vi "OCR Check(Center & Left).vi"(8 "error in (no error)":errorcluster, 11 "Image Path":path=path "C:/images/img1.jpeg") -> (0 "error out":errorcluster, 1 "Image Out":T2(plugin-control), 2 "RIGHT":bool, 3 "OCR Check":T3={"C_Center"="6 G D 6 4 8 6", "Center 2"=TRUE, "C_Top"="8 G D 6 4 8 6", "Top 2"=TRUE, "C_Bottom"="6 G D 6 4 4 8", "Bottom 2"=TRUE, "RH_TOP"="", "Top_RH"=FALSE, "RH_CENTER"="", "Center_RH"=FALSE, "RH_BOTTOM"="6 G D 6 4 8 6", "Bottom_RH"=TRUE}, 7 "Pattern Presence":bool)   [LabVIEW 2019]
panel:
  out "OCR 3 Digit":T1
  out "CENTER":bool
  out "Read bottom":string
  out "Read Center":string caption="Read String"
  out "Read Top":string
  out "y":sgl=319.5874
  out "x":sgl=660.16455
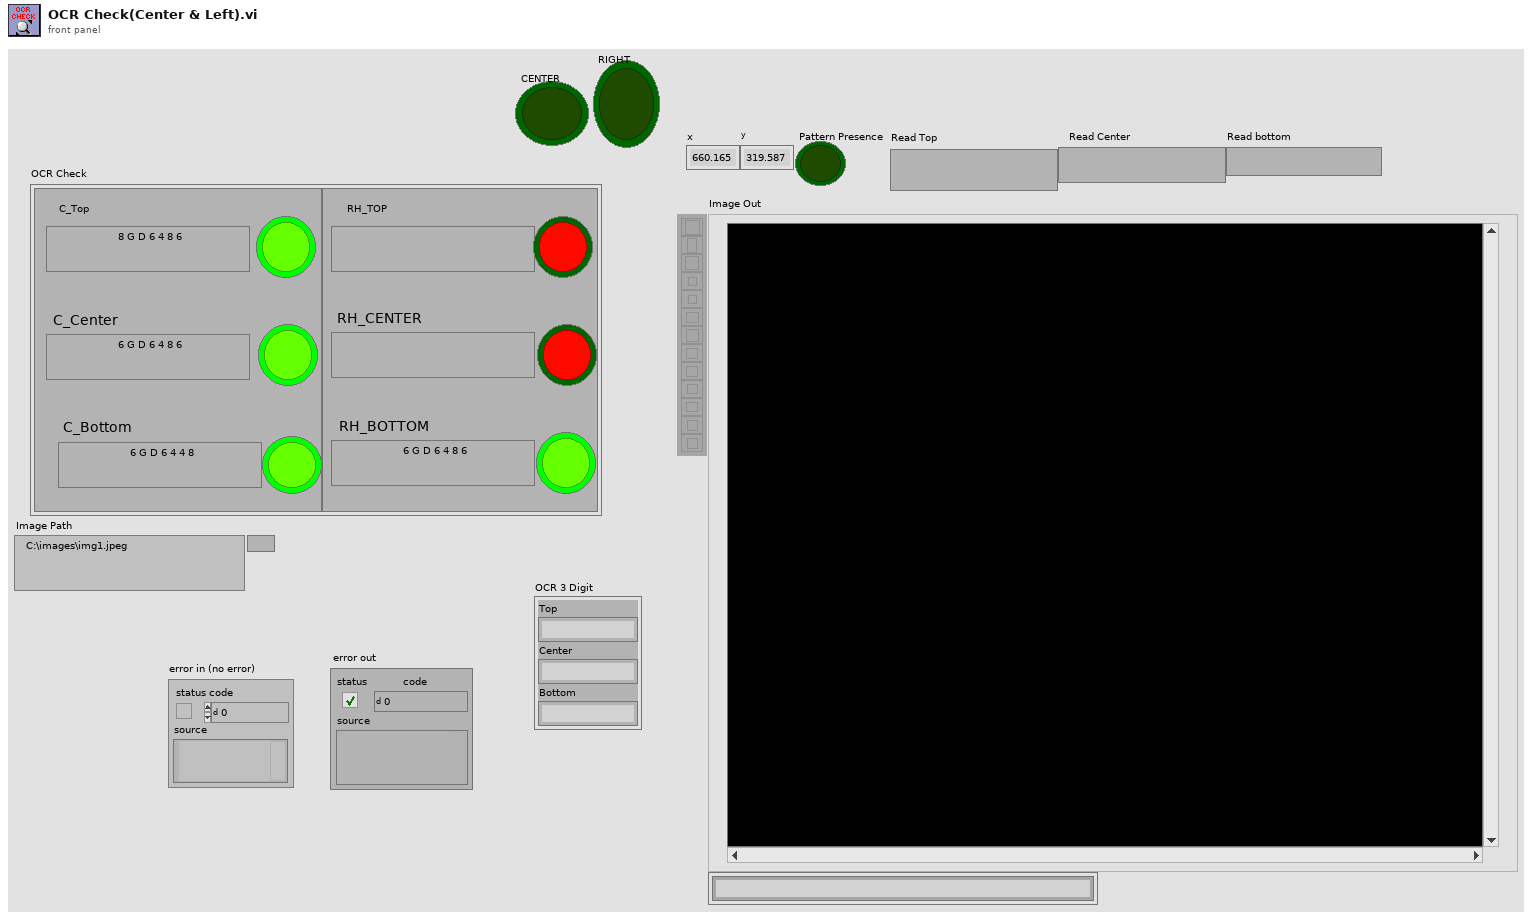
[diagram p1: front panel]
types:
  T1 = cluster{"Top":string, "Center":string, "Bottom":string}
  T2 = typedef "IMAQ Image.ctl" = refnum<image>
  T3 = cluster{"C_Center":string, "Center 2":bool, "C_Top":string, "Top 2":bool, "C_Bottom":string, "Bottom 2":bool, "RH_TOP":string, "Top_RH":bool, "RH_CENTER":string, "Center_RH":bool, "RH_BOTTOM":string, "Bottom_RH":bool}
  T4 = cluster{"Center":string, "Center 2":bool, "Top":string, "Top 2":bool, "Bottom":string, "Bottom 2":bool, "RH_TOP":string, "Top_RH":bool, "RH_CENTER":string, "Center_RH":bool, "RH_BOTTOM":string, "Bottom_RH":bool}
  T5 = typedef "Image Type" = u32
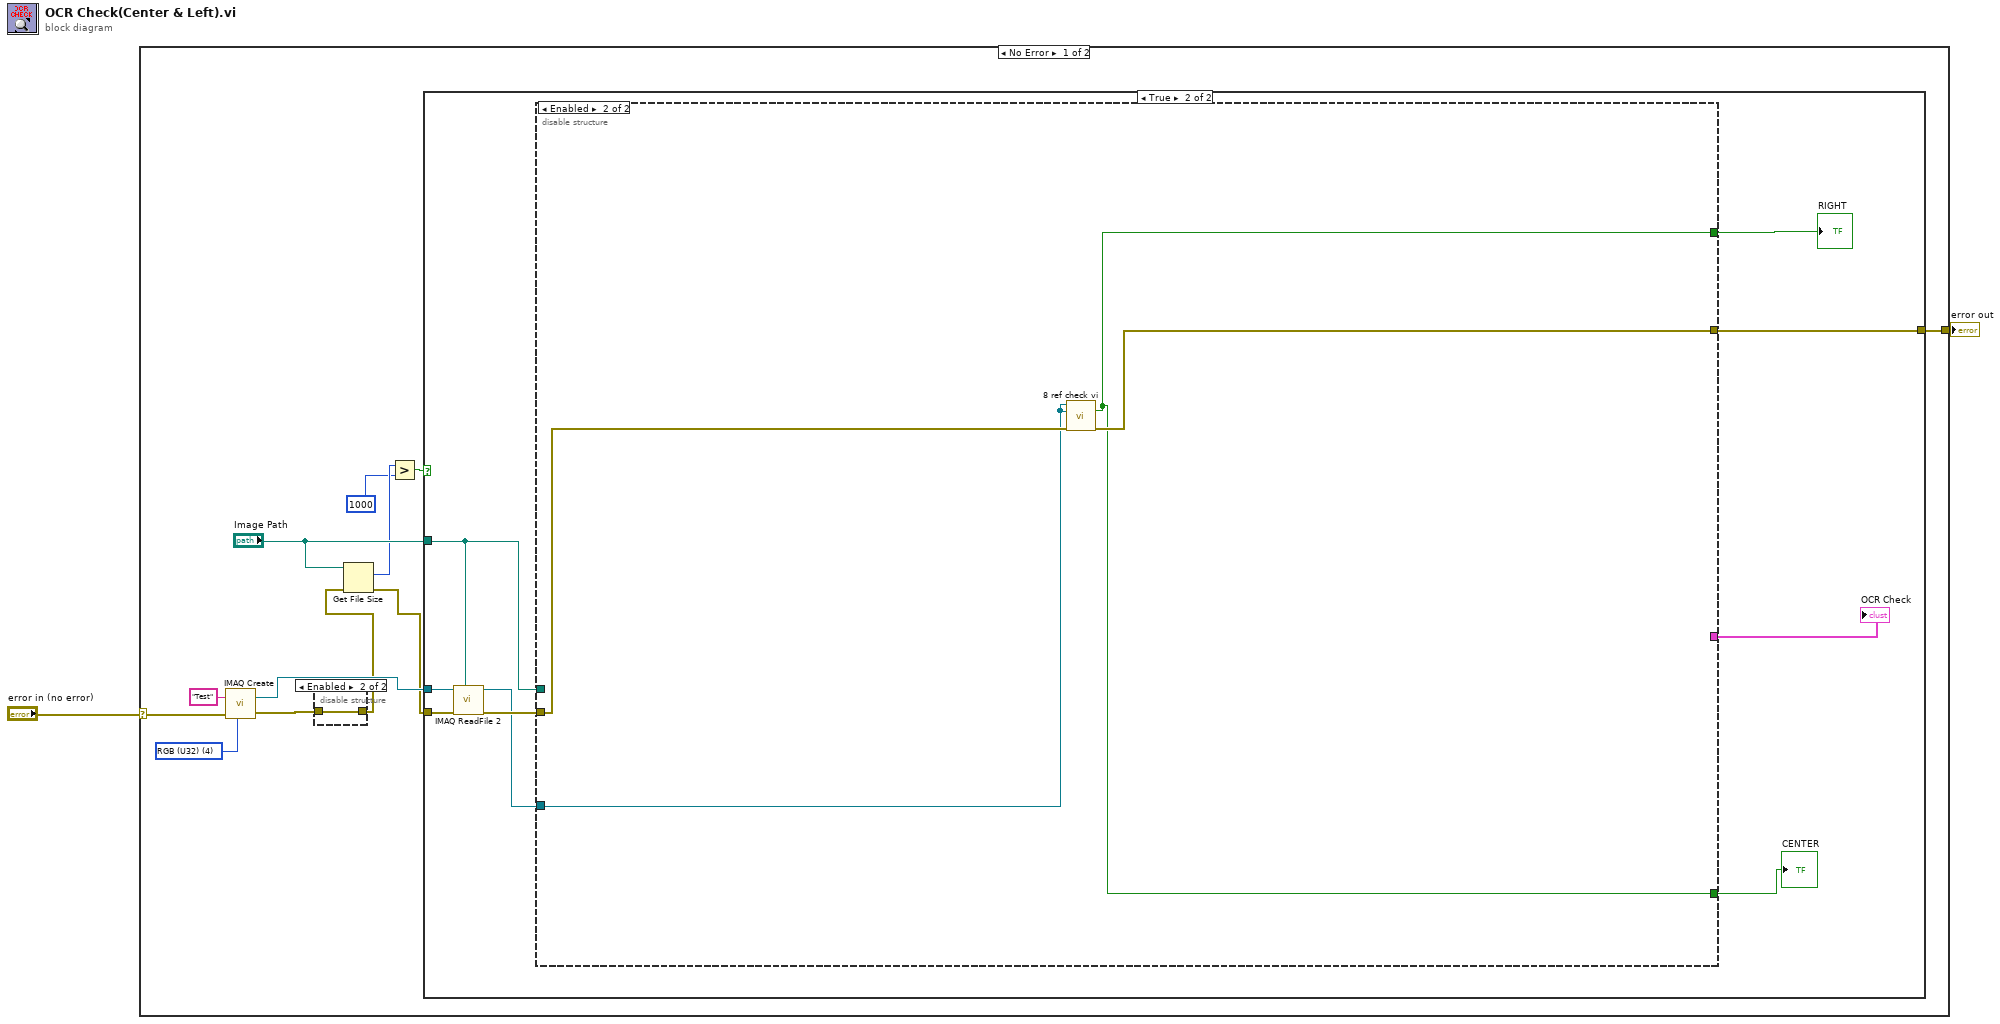
[diagram p0: block diagram]
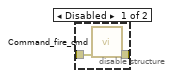
[diagram p2: hidden frame]
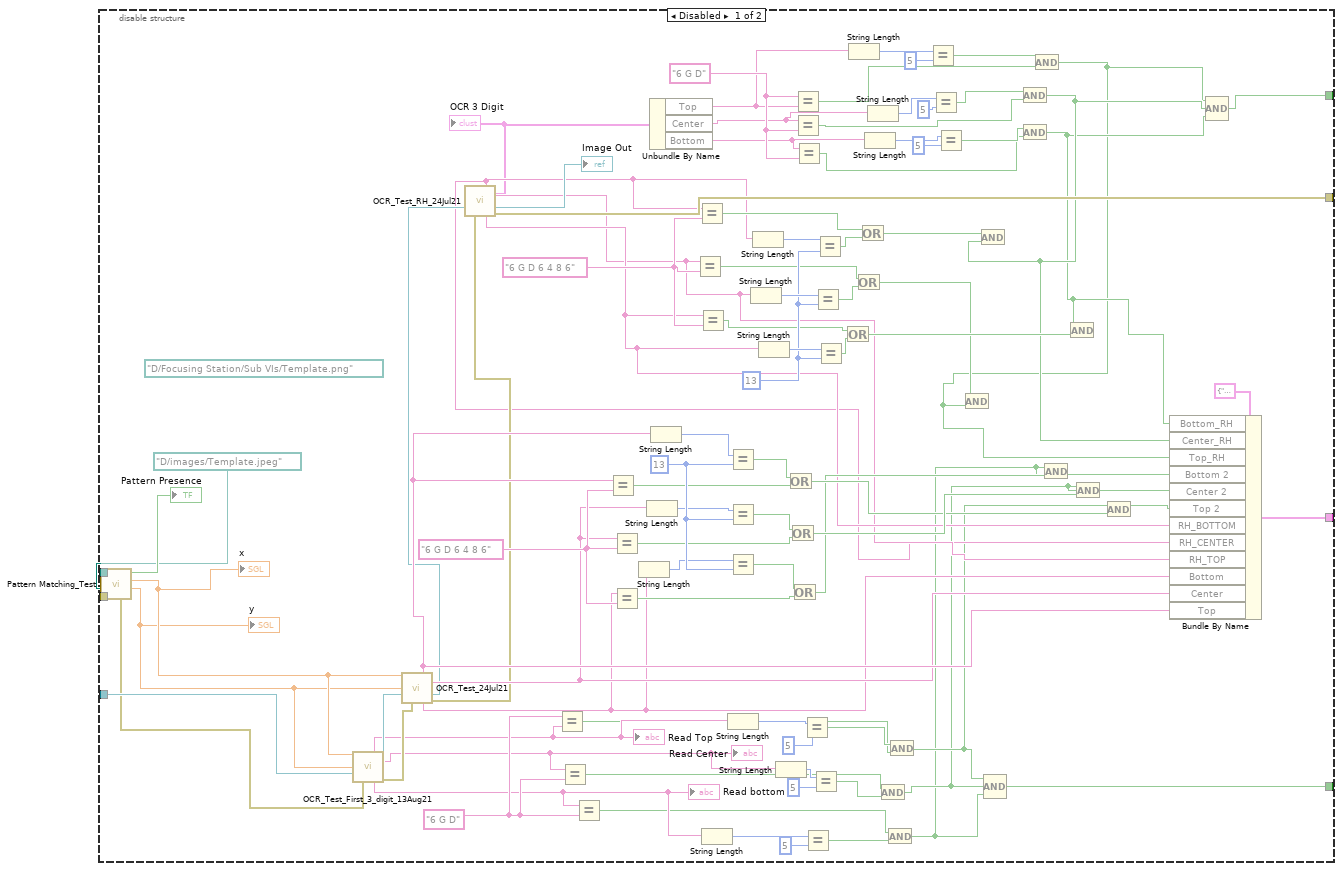
[diagram p4: hidden frame]
diagram:
  n1 = case shown="No Error" "error in (no error)" {
    selector: "error in (no error)" -> [w3 w123]
    tunnel: [w4 w123] -> w2
    frame No Error {
      w12 = T5 4 items=["Grayscale (U8)", "Grayscale (I16)", "Grayscale (SGL)", "Complex (CSG)", "RGB (U32)", "HSL (U32)", "RGB (U64)", "Grayscale (U16)"] ("Image Type")
      n2 = call "IMAQ Create"("Image Name"="Test", "Image Type"=w12, "error in (no error)"=w3) -> ("New Image"=w14:T2, "error out"=w11:errorcluster)  [unwired: 2 in]
      n3 = disable-structure shown="Enabled" {
        disable-tunnel: w11 -> [w16 w17]
        disable-tunnel: [w15 w17] -> w8
        frame Disabled {
          n4 = call "Command_fire_cmd.vi"("error in"=w16) -> ("error out"=w15:errorcluster)  [unwired: 6 in, 2 out]
        }
        frame Enabled {
        }
      }
      n5 = Get File Size(file="Image Path", error in=w8) -> (size (in bytes)=w7:i64, 0:w9:errorcluster)  [unwired: 1 out]
      n6 = Greater?(x=w7, y=i64 1000) -> (0:w5:bool)
      n7 = case shown="True" w5 {
        tunnel: w14 -> [_ w26]
        tunnel: "Image Path" -> [_ w24]
        tunnel: w9 -> [w18 w23]
        tunnel: [w18 w22] -> w4
        frame False {
        }
        frame True {
          n8 = call "IMAQ ReadFile 2"("File Path"=w24, "error in (no error)"=w23, "Image"=w26) -> ("error out"=w25:errorcluster, "Image Out"=w21:T2)  [unwired: 4 in, 3 out]
          n9 = disable-structure shown="Enabled" {
            disable-tunnel: [w87 _] -> w27
            disable-tunnel: w25 -> [w83 w121]
            disable-tunnel: w24 -> [w82 _]
            disable-tunnel: [w80 w122] -> w22
            disable-tunnel: w21 -> [w72 w119]
            disable-tunnel: [w29 w120] -> w20
            disable-tunnel: [w28 w120] -> w19
            frame Disabled {
              (unwired) path "D:/Focusing Station/Sub VIs/Template.png" ("Image File Path")
              w51 = "6 G D" ("y")
              w68 = "6 G D" ("y")
              w103 = 13
              w117 = 13 ("y")
              w104 = "6 G D 6 4 8 6" ("y")
              w118 = "6 G D 6 4 8 6" ("y")
              n10 = call "Pattern Matching_Test.vi"("error in (no error)"=w83, "Template file path"=path "D:/images/Template.jpeg" ("Image File Path"), "File Path"=w82) -> ("y"=w73:sgl, "x"=w74:sgl, "Pattern Presence"=→"Pattern Presence":bool, "error out"=w70:errorcluster)  [unwired: 4 in, 1 out]
              "x" <- w74
              "y" <- w73
              n11 = call "OCR_Test_First_3_digit_13Aug21.vi"("x"=w74, "y"=w73, "Image in"=w72, "error in (no error)"=w70) -> ("Read Top"=w66:string, "Read Center"=w65:string, "Image"=w71:T2, "Read bottom"=w67:string, "error out"=w69:errorcluster)  [unwired: 7 in]
              "Read Top" <- w66
              "Read Center" <- w65
              "Read bottom" <- w67
              n12 = call "OCR_Test_24Jul21.vi"("x"=w74, "y"=w73, "Image in"=w71, "error in (no error)"=w69) -> ("Read Top"=w102:string, "Read Center"=w101:string, "Image"=w85:T2, "Read bottom"=w100:string, "error out"=w84:errorcluster)  [unwired: 7 in]
              n13 = call "OCR_Test_RH_24Jul21.vi"("Image in"=w85, "error in (no error)"=w84) -> ("OCR 3 Digit"=w52:T1, "Read Center"=w77:string, "Read Top"=w78:string, "Image"=→"Image Out":T2, "Read bottom"=w96:string, "error out"=w80:errorcluster)  [unwired: 8 in]
              "OCR 3 Digit" <- w52
              n14 = Equal?(x=w68, y=w66) -> (x = y?=w57:bool)
              n15 = Equal?(x=w65, y=w68) -> (x = y?=w54:bool)
              n16 = Equal?(x=w67, y=w68) -> (x = y?=w56:bool)
              n17 = Equal?(x=w102, y=w118) -> (x = y?=w116:bool)
              n18 = Equal?(x=w101, y=w118) -> (x = y?=w111:bool)
              n19 = Equal?(x=w100, y=w118) -> (x = y?=w110:bool)
              n20 = String Length(string=w100) -> (length=w112:i32)
              n21 = String Length(string=w101) -> (length=w113:i32)
              n22 = Unbundle By Name(w52) -> ("Top"=w50:string, "Center"=w49:string, "Bottom"=w48:string)
              n23 = String Length(string=w102) -> (length=w114:i32)
              n24 = Equal?(x=w78, y=w104) -> (x = y?=w93:bool)
              n25 = Equal?(x=w77, y=w104) -> (x = y?=w94:bool)
              n26 = Equal?(x=w96, y=w104) -> (x = y?=w91:bool)
              n27 = String Length(string=w67) -> (length=w64:i32)
              n28 = Equal?(x=w114, y=w117) -> (x = y?=w115:bool)
              n29 = Equal?(x=w113, y=w117) -> (x = y?=w108:bool)
              n30 = Equal?(x=w112, y=w117) -> (x = y?=w109:bool)
              n31 = String Length(string=w66) -> (length=w61:i32)
              n32 = String Length(string=w78) -> (length=w106:i32)
              n33 = String Length(string=w77) -> (length=w107:i32)
              n34 = String Length(string=w96) -> (length=w105:i32)
              n35 = String Length(string=w65) -> (length=w62:i32)
              n36 = Or(x=w115, y=w116) -> (x .or. y?=w98:bool)
              n37 = Or(x=w108, y=w111) -> (x .or. y?=w99:bool)
              n38 = Or(x=w109, y=w110) -> (x .or. y?=w97:bool)
              n39 = Equal?(x=w51, y=w50) -> (x = y?=w40:bool)
              n40 = Equal?(x=w49, y=w51) -> (x = y?=w38:bool)
              n41 = Equal?(x=w48, y=w51) -> (x = y?=w36:bool)
              n42 = Equal?(x=w61, y=5) -> (x = y?=w58:bool)
              n43 = Equal?(x=w64, y=5) -> (x = y?=w55:bool)
              n44 = Equal?(x=w62, y=5) -> (x = y?=w53:bool)
              n45 = Equal?(x=w106, y=w103) -> (x = y?=w92:bool)
              n46 = Equal?(x=w107, y=w103) -> (x = y?=w95:bool)
              n47 = Equal?(x=w105, y=w103) -> (x = y?=w90:bool)
              n48 = Or(x=w91, y=w90) -> (x .or. y?=w89:bool)
              n49 = String Length(string=w50) -> (length=w47:i32)
              n50 = Or(x=w93, y=w92) -> (x .or. y?=w75:bool)
              n51 = Or(x=w94, y=w95) -> (x .or. y?=w76:bool)
              n52 = String Length(string=w48) -> (length=w45:i32)
              n53 = String Length(string=w49) -> (length=w46:i32)
              n54 = And(x=w54, y=w53) -> (x .and. y?=w31:bool)
              n55 = And(x=w56, y=w55) -> (x .and. y?=w30:bool)
              n56 = And(x=w58, y=w57) -> (x .and. y?=w32:bool)
              n57 = Equal?(x=w47, y=5) -> (x = y?=w41:bool)
              n58 = Equal?(x=w46, y=5) -> (x = y?=w39:bool)
              n59 = Equal?(x=w45, y=5) -> (x = y?=w37:bool)
              n60 = Compound Arithmetic op=AND(w32, w31, w30) -> (w28:bool)
              n61 = And(x=w39, y=w38) -> (x .and. y?=w35:bool)
              n62 = And(x=w76, y=w35) -> ()  [unwired: 1 out]
              n63 = And(x=w37, y=w36) -> (x .and. y?=w34:bool)
              n64 = And(x=w41, y=w40) -> (x .and. y?=w33:bool)
              n65 = And(x=w75, y=w33) -> ()  [unwired: 1 out]
              n66 = And(x=w30, y=w97) -> ()  [unwired: 1 out]
              n67 = And(x=w34, y=w89) -> ()  [unwired: 1 out]
              n68 = And(x=w31, y=w99) -> ()  [unwired: 1 out]
              n69 = And(x=w32, y=w98) -> ()  [unwired: 1 out]
              n70 = Bundle By Name(cluster=T4 {"Center"="", "Center 2"=FALSE, "Top"="", "Top 2"=FALSE, "Bottom"="", "Bottom 2"=FALSE, "RH_TOP"="", "Top_RH"=FALSE, "RH_CENTER"="", "Center_RH"=FALSE, "RH_BOTTOM"="", "Bottom_RH"=FALSE} ("output cluster"), "Bottom_RH"=w34, "Center_RH"=w35, "Top_RH"=w33, "Bottom 2"=w30, "Center 2"=w31, "Top 2"=w32, "RH_BOTTOM"=w96, "RH_CENTER"=w77, "RH_TOP"=w78, "Bottom"=w100, "Center"=w101, "Top"=w102) -> (w87:T4)
              n71 = Compound Arithmetic op=AND(w33, w35, w34) -> (w29:bool)
            }
            frame Enabled {
              n72 = call "8 ref check vi.vi"("Image In"=w119, "Image Dst"=w119, "error in"=w121) -> ("x = y?"=w120:bool, "error out"=w122:errorcluster)  [unwired: 9 in, 2 out]
            }
          }
          "OCR Check" <- w27
          "RIGHT" <- w20
          "CENTER" <- w19
        }
      }
    }
    frame Error {
    }
  }
  "error out" <- w2
